vi "FPGA-1900 Motor Automation Test.vi"() -> ()   [LabVIEW 2014]
uses:
  <vilib>/robotics/Utilities/Encoder Count Encoding.ctl
  <vilib>/rvi/Emulation/niFpgaGetClockAttributes.vi
  <vilib>/rvi/Emulation/niFpgaSctlEmulationGetInTimedLoop.vi
  <vilib>/rvi/Emulation/niFpgaEmulationReportErrorSimple.vi
  <vilib>/rvi/Emulation/niFpgaProcessEmulError.vi
  <vilib>/robotics/Utilities/FPGA Utilities/Generate Digital Pulse (uSec).vi
  <vilib>/rvi/Emulation/niFpgaCriticalErrorInLSC.vi
  <vilib>/robotics/Utilities/FPGA Utilities/Count Two Phase Digital Encoder.vi
  <instrlib>/Devantech SRF05/FPGA/Read Distance (Mode 1).vi
  <vilib>/robotics/Utilities/FPGA Utilities/NI_Robotics_FPGA Utilities.lvlib
  <vilib>/robotics/Utilities/NI_Robotics Utilities.lvlib
  <instrlib>/Devantech SRF05/FPGA/NI_Robotics_Devantech SRF05 (FPGA).lvlib
panel:
  in  "Stop motors":bool
  in  "Smart Stop":bool
  out "Move Stop":bool
  in  "Right Count Length":i16
  in  "Left Count Length":i16
  out "Centre Left Dist (cm)":fxp<+,24,16>=95.46875
  out "Front Left Dist (cm)":fxp<+,24,16>=20.84375
  out "Front Right Dist (cm)":fxp<+,24,16>=20.43359375
  in  "Belt 1 Dir":bool
  in  "Belt 2 Dir":bool
  in  "Stop Belt 1":bool=TRUE
  in  "Stop Belt 2":bool=TRUE
  in  "Belt 2 pulse width (uSec)":u32=1000
  in  "Belt 1 pulse width (uSec)":u32=1000
  in  "Stop Right":bool=TRUE
  out "Centre Right Dist (cm)":fxp<+,24,16>=61.78125
  out "Left Wheel":i32
  out "Right Wheel":i32
  in  "reset wheel count (T)":bool
  in  "Right motor pulse width (uSec)":u32=100
  in  "Left motor pulse width (uSec)":u32=100
  in  "Stop Left":bool=TRUE
  in  "Right Motor":bool=TRUE
  in  "Left Motor":bool=TRUE
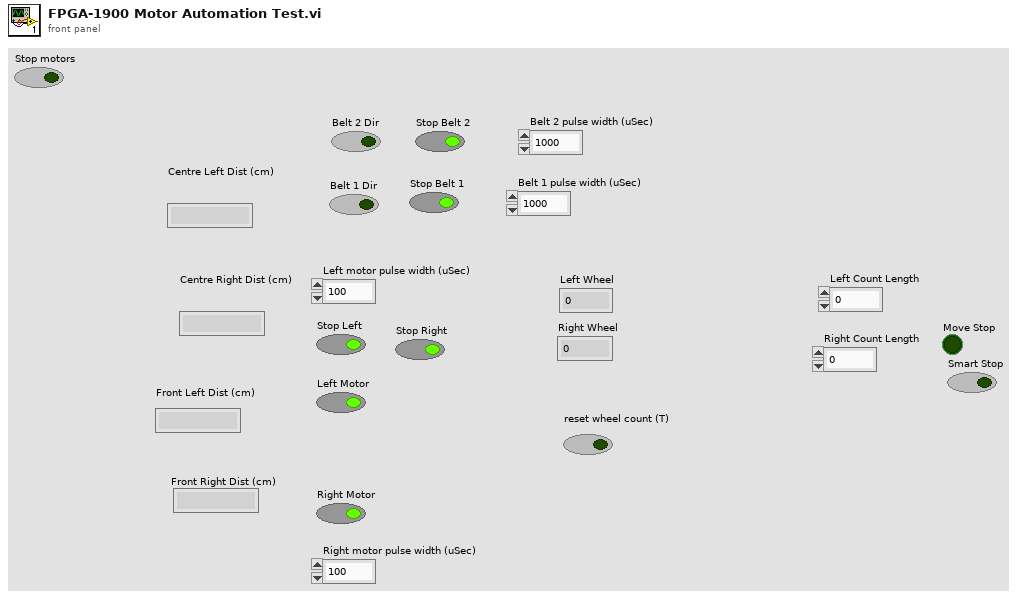
[diagram p1: front panel]
types:
  T1 = typedef "NI_Robotics Utilities.lvlib/Encoder Count Encoding.ctl" = enum16{"X1", "X2", "X4"}
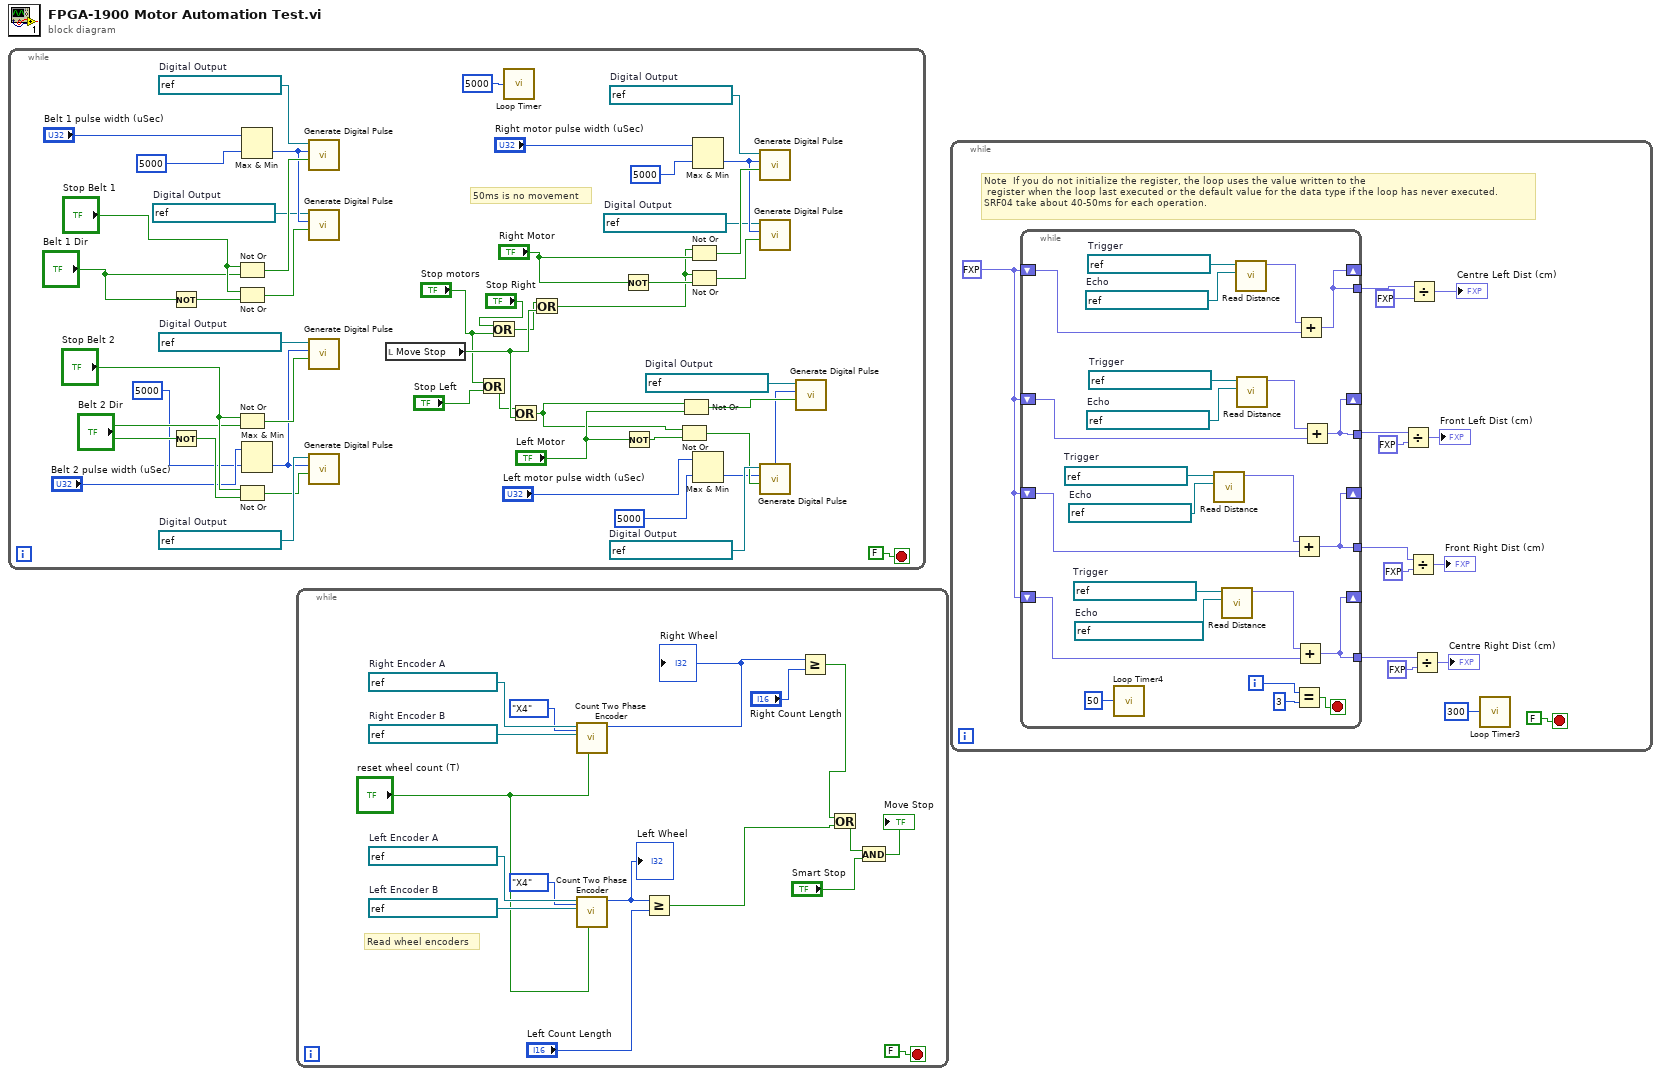
[diagram p0: block diagram]
diagram:
  n1 = while {
    stop <- FALSE stop-if-true
    w28 = refnum<k21> "ConnectorC/DIO7"  # Digital Output
    w27 = refnum<k21> "ConnectorC/DIO6"  # Digital Output
    w17 = refnum<k21> "ConnectorC/DIO5"  # Digital Output
    w15 = refnum<k21> "ConnectorC/DIO4"  # Digital Output
    w48 = refnum<k21> "ConnectorC/DIO3"  # Digital Output
    w47 = refnum<k21> "ConnectorC/DIO2"  # Digital Output
    w35 = refnum<k21> "ConnectorC/DIO1"  # Digital Output
    w33 = refnum<k21> "ConnectorC/DIO0"  # Digital Output
    # "50ms is no movement"
    n2 = Not(x="Belt 1 Dir") -> (.not. x?=w26:bool)
    n3 = Not(x="Belt 2 Dir") -> (.not. x?=w21:bool)
    n4 = Not Or(1:"Belt 1 Dir", 2:"Stop Belt 1") -> (0:w24:bool)
    n5 = Not Or(1:w26, 2:"Stop Belt 1") -> (0:w25:bool)
    n6 = Not Or(1:"Belt 2 Dir", 2:"Stop Belt 2") -> (0:w23:bool)
    n7 = Not Or(1:w21, 2:"Stop Belt 2") -> (0:w22:bool)
    n8 = Max & Min(x="Belt 1 pulse width (uSec)", y=u32 5000 ("Motor period (uSec)")) -> (min(x,y)=w18:u32)  [unwired: 1 out]
    n9 = Max & Min(x="Belt 2 pulse width (uSec)", y=u32 5000 ("Motor period (uSec)")) -> (min(x,y)=w19:u32)  [unwired: 1 out]
    n10 = call-poly <vilib>:"Generate Digital Pulse.vi"("invert pulse (F)"=w24, "pulse width (uSec)"=w18, "FPGA digital output"=w15) -> ()  [unwired: 9 in]
    n11 = call-poly <vilib>:"Generate Digital Pulse.vi"("invert pulse (F)"=w25, "pulse width (uSec)"=w18, "FPGA digital output"=w17) -> ()  [unwired: 9 in]
    n12 = call-poly <vilib>:"Generate Digital Pulse.vi"("invert pulse (F)"=w23, "pulse width (uSec)"=w19, "FPGA digital output"=w27) -> ()  [unwired: 9 in]
    n13 = call-poly <vilib>:"Generate Digital Pulse.vi"("invert pulse (F)"=w22, "pulse width (uSec)"=w19, "FPGA digital output"=w28) -> ()  [unwired: 9 in]
    n14 = local read "Move Stop"() -> (w6:bool)
    n15 = Or(x="Stop motors", y="Stop Left") -> (x .or. y?=w1:bool)
    n16 = Or(x="Stop Right", y="Stop motors") -> (x .or. y?=w2:bool)
    n17 = call "Loop Timer"("Count(uSec)"=u32 5000) -> ()  [unwired: 1 out]
    n18 = Or(x=w1, y=w6) -> (x .or. y?=w9:bool)
    n19 = Or(x=w2, y=w6) -> (x .or. y?=w10:bool)
    n20 = Not(x="Right Motor") -> (.not. x?=w45:bool)
    n21 = Not(x="Left Motor") -> (.not. x?=w39:bool)
    n22 = Not Or(1:w39, 2:w9) -> (0:w40:bool)
    n23 = Not Or(1:"Left Motor", 2:w9) -> (0:w41:bool)
    n24 = Not Or(1:"Right Motor", 2:w10) -> (0:w43:bool)
    n25 = Not Or(1:w45, 2:w10) -> (0:w44:bool)
    n26 = Max & Min(x="Right motor pulse width (uSec)", y=u32 5000 ("Left motor pulse period (uSec)")) -> (min(x,y)=w36:u32)  [unwired: 1 out]
    n27 = Max & Min(x="Left motor pulse width (uSec)", y=u32 5000 ("Left motor pulse period (uSec)")) -> (min(x,y)=w37:u32)  [unwired: 1 out]
    n28 = call-poly <vilib>:"Generate Digital Pulse.vi"("invert pulse (F)"=w43, "pulse width (uSec)"=w36, "FPGA digital output"=w33) -> ()  [unwired: 9 in]
    n29 = call-poly <vilib>:"Generate Digital Pulse.vi"("invert pulse (F)"=w44, "pulse width (uSec)"=w36, "FPGA digital output"=w35) -> ()  [unwired: 9 in]
    n30 = call-poly <vilib>:"Generate Digital Pulse.vi"("invert pulse (F)"=w40, "pulse width (uSec)"=w37, "FPGA digital output"=w48) -> ()  [unwired: 9 in]
    n31 = call-poly <vilib>:"Generate Digital Pulse.vi"("invert pulse (F)"=w41, "pulse width (uSec)"=w37, "FPGA digital output"=w47) -> ()  [unwired: 9 in]
  }
  n32 = while "Encoder Loop" {
    stop <- FALSE stop-if-true
    w61 = refnum<k21> "ConnectorA/DIO15"  # Right Encoder B
    w62 = refnum<k21> "ConnectorA/DIO14"  # Right Encoder A
    w63 = refnum<k21> "ConnectorA/DIO12"  # Left Encoder B
    w64 = refnum<k21> "ConnectorA/DIO11"  # Left Encoder A
    # "Read wheel encoders"
    n33 = call-poly <vilib>:"Count Two Phase Encoder.vi"("reset (F)"="reset wheel count (T)", "count encoding (X1)"=Encoder_Count_Encoding."X4" ("count multiplier (X1)"), "phase B FPGA digital input"=w61, "phase A FPGA digital input"=w62) -> ("new count"=w49:i32)  [unwired: 6 in, 1 out]
    "Right Wheel" <- w49
    n34 = call-poly <vilib>:"Count Two Phase Encoder.vi"("reset (F)"="reset wheel count (T)", "count encoding (X1)"=Encoder_Count_Encoding."X4" ("count multiplier (X1)"), "phase B FPGA digital input"=w63, "phase A FPGA digital input"=w64) -> ("new count"=w59:i32)  [unwired: 6 in, 1 out]
    "Left Wheel" <- w59
    n35 = Greater Or Equal?(x=w59, y="Left Count Length") -> (x >= y?=w51:bool)
    n36 = Greater Or Equal?(x=w49, y="Right Count Length") -> (x >= y?=w55:bool)
    n37 = Or(x=w55, y=w51) -> (x .or. y?=w53:bool)
    n38 = And(x=w53, y="Smart Stop") -> (x .and. y?=→"Move Stop":bool)
  }
  n39 = while {
    stop <- FALSE stop-if-true
    w68 = fxp<+/-,32,16> 0.0
    # "Note  If you do not initialize the register, the loop uses the value written to the\n register when the loop last executed or the default value for the data type if the loop has never executed.\nSRF04 take about 40-50ms for each operation."
    n40 = while {
      tunnel: [w82] -> w77
      shift-right: [w82] -> _
      shift-left: w68 -> [w81]
      shift-right: [w85] -> _
      shift-left: w68 -> [w84]
      tunnel: [w85] -> w74
      shift-right: [w88] -> _
      shift-left: w68 -> [w87]
      tunnel: [w88] -> w72
      shift-right: [w90] -> _
      shift-left: w68 -> [w92]
      tunnel: [w90] -> w69
      i -> [w100]
      stop <- w101 stop-if-true
      w93 = refnum<k21> "ConnectorA/DIO1"  # Echo
      w94 = refnum<k21> "ConnectorA/DIO2"  # Trigger
      w95 = refnum<k21> "ConnectorA/DIO5"  # Echo
      w96 = refnum<k21> "ConnectorA/DIO6"  # Trigger
      w97 = refnum<k21> "ConnectorA/DIO3"  # Echo
      w98 = refnum<k21> "ConnectorA/DIO4"  # Trigger
      w103 = refnum<k21> "ConnectorA/DIO13"  # Echo
      w104 = refnum<k21> "ConnectorA/DIO0"  # Trigger
      n41 = call "Loop Timer4"("Count(mSec)"=u32 50 ("Count(uSec)")) -> ()  [unwired: 1 out]
      n42 = call-poly <instrlib>:"Read Distance.vi"("echo line"=w97, "trigger line"=w98) -> ("distance (cm)"=w86:fxp<+,24,16>)  [unwired: 8 in, 1 out]
      n43 = call-poly <instrlib>:"Read Distance.vi"("echo line"=w103, "trigger line"=w104) -> ("distance (cm)"=w83:fxp<+,24,16>)  [unwired: 8 in, 1 out]
      n44 = call-poly <instrlib>:"Read Distance.vi"("echo line"=w93, "trigger line"=w94) -> ("distance (cm)"=w91:fxp<+,24,16>)  [unwired: 8 in, 1 out]
      n45 = call-poly <instrlib>:"Read Distance.vi"("echo line"=w95, "trigger line"=w96) -> ("distance (cm)"=w89:fxp<+,24,16>)  [unwired: 8 in, 1 out]
      n46 = Add(x=w86, y=w84) -> (x+y=w85:fxp<+/-,32,16>)
      n47 = Equal?(x=w100, y=3) -> (x = y?=w101:bool)
      n48 = Add(x=w83, y=w81) -> (x+y=w82:fxp<+/-,32,16>)
      n49 = Add(x=w91, y=w92) -> (x+y=w90:fxp<+/-,32,16>)
      n50 = Add(x=w89, y=w87) -> (x+y=w88:fxp<+/-,32,16>)
    }
    n51 = Divide(x=w72, y=fxp<+,25,17> 3.0) -> (x/y=→"Front Left Dist (cm)":fxp<+/-,57,24>)
    n52 = Divide(x=w74, y=fxp<+,25,17> 3.0) -> (x/y=→"Front Right Dist (cm)":fxp<+/-,57,24>)
    n53 = Divide(x=w69, y=fxp<+,25,17> 3.0) -> (x/y=→"Centre Left Dist (cm)":fxp<+/-,57,24>)
    n54 = Divide(x=w77, y=fxp<+,25,17> 3.0) -> (x/y=→"Centre Right Dist (cm)":fxp<+/-,57,24>)
    n55 = call "Loop Timer3"("Count(uSec)"=u32 300) -> ()  [unwired: 1 out]
  }
